vi "_FPGA Toggle Electronics.vi"(5 "error in":errorcluster, 7 "Ele On (1 for ON and 0 for OFF)":u32) -> (0 "error out":errorcluster)   [LabVIEW 2012]
uses:
  Type/_FPGA Indicator.ctl
  _RT Global.vi
  <vilib>/Utility/error.llb/Error Cluster From Error Code.vi
  <vilib>/rvi/errors/niLvFpgaAdjustHostInterfaceError.vi
  <vilib>/rvi/interface/nirviReadWriteControl/nirviReadWriteControl.xnode
  FPGA Bitfiles/FPGA9602.lvbitx
  NiFpgaLv.dll
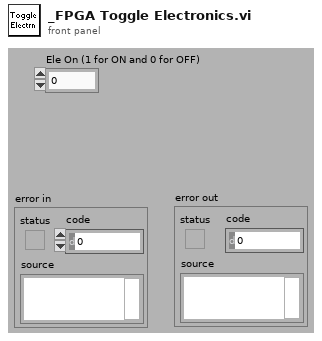
[diagram p1: front panel]
types:
  T1 = typedef "Semaphore RefNum" = refnum<k1>
  T2 = typedef "_FPGA Indicator.ctl" = enum16{"Done", "Ready", "Count Available", "SendSerial", "LED State"}
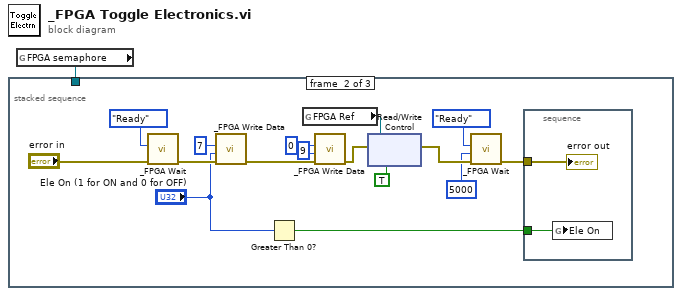
[diagram p0: block diagram]
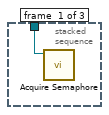
[diagram p2: hidden frame]
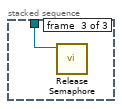
[diagram p3: hidden frame]
diagram:
  n1 = global read "_RT Global.vi" "FPGA semaphore"() -> (w1:T1)
  n2 = stacked-sequence {
    tunnel: w1 -> [w2 _ w21]
    frame #0 {
      n3 = call <vilib>:"Acquire Semaphore.vi"("semaphore"=w2) -> ()  [unwired: 2 in, 5 out]
    }
    frame #1 {
      n4 = call "_FPGA Wait.vi"("error in"="error in", "Indicator"=_FPGA_Indicator."Ready") -> ("error out"=w9:errorcluster)  [unwired: 3 in, 2 out]
      n5 = call "_FPGA Write Data.vi"("error in"=w9, "Data"="Ele On (1 for ON and 0 for OFF)", "Address"=u16 7) -> ("error out"=w7:errorcluster)  [unwired: 3 in, 2 out]
      n6 = Greater Than 0?(x="Ele On (1 for ON and 0 for OFF)") -> (x > 0?=w5:bool)
      n7 = global read "_RT Global.vi" "FPGA Ref"() -> (w3:refnum<k20>)
      n8 = call "_FPGA Write Data.vi"("error in"=w7, "Data"=u32 9 ("Address"), "Address"=u16 0) -> ("error out"=w17:errorcluster)  [unwired: 3 in, 2 out]
      n9 = xnode "Read/Write Control"("FPGA VI Reference In"=w3, "error in"=w17, "Start"=TRUE) -> ("error out"=w12:errorcluster)  [unwired: 1 out]
      n10 = call "_FPGA Wait.vi"("error in"=w12, "Timeout (2000ms)"=u32 5000, "Indicator"=_FPGA_Indicator."Ready") -> ("error out"=w8:errorcluster)  [unwired: 2 in, 2 out]
      n11 = stacked-sequence {
        tunnel: w8 -> [w20]
        tunnel: w5 -> [w19]
        frame #0 {
          n12 = global write "_RT Global.vi" "Ele On"(w19) -> ()
          "error out" <- w20
        }
      }
    }
    frame #2 {
      n13 = call <vilib>:"Release Semaphore.vi"("semaphore"=w21) -> ()  [unwired: 1 in, 6 out]
    }
  }
